vi "decade-down-counter.vi"() -> ()   [LabVIEW 2021]
uses:
  4-bit-disp.ctl
  7-segment-display.ctl
  !4-bit-cont.ctl
panel:
  out "7-segment":T1
  out "Iteration":i32
  out "!4-bit-display":T2
  out "4-bit-display":T3
  in  "Stop Button":bool
  in  "CLK":bool
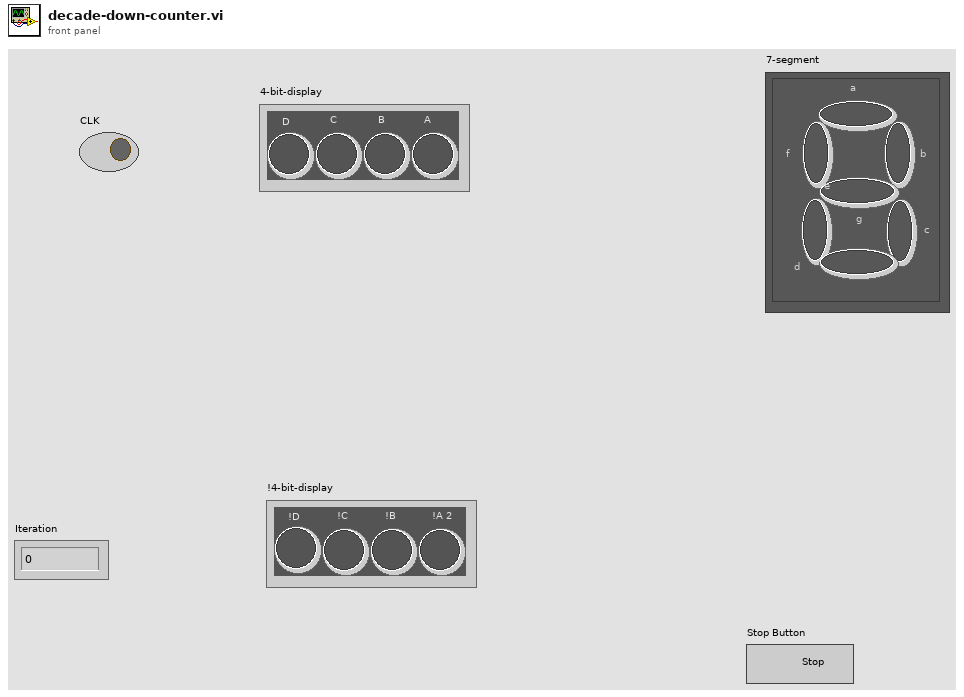
[diagram p1: front panel]
types:
  T1 = typedef "7-segment-display.ctl" = cluster{"a":bool, "b":bool, "c":bool, "d":bool, "e":bool, "f":bool, "g":bool}
  T2 = cluster{"!D":bool, "!C":bool, "!B":bool, "!A 2":bool}
  T3 = typedef "4-bit-disp.ctl" = cluster{"D":bool, "C":bool, "B":bool, "A":bool}
  T4 = typedef "!4-bit-cont.ctl" = cluster{"!D":bool, "!C":bool, "!B":bool, "!A":bool}
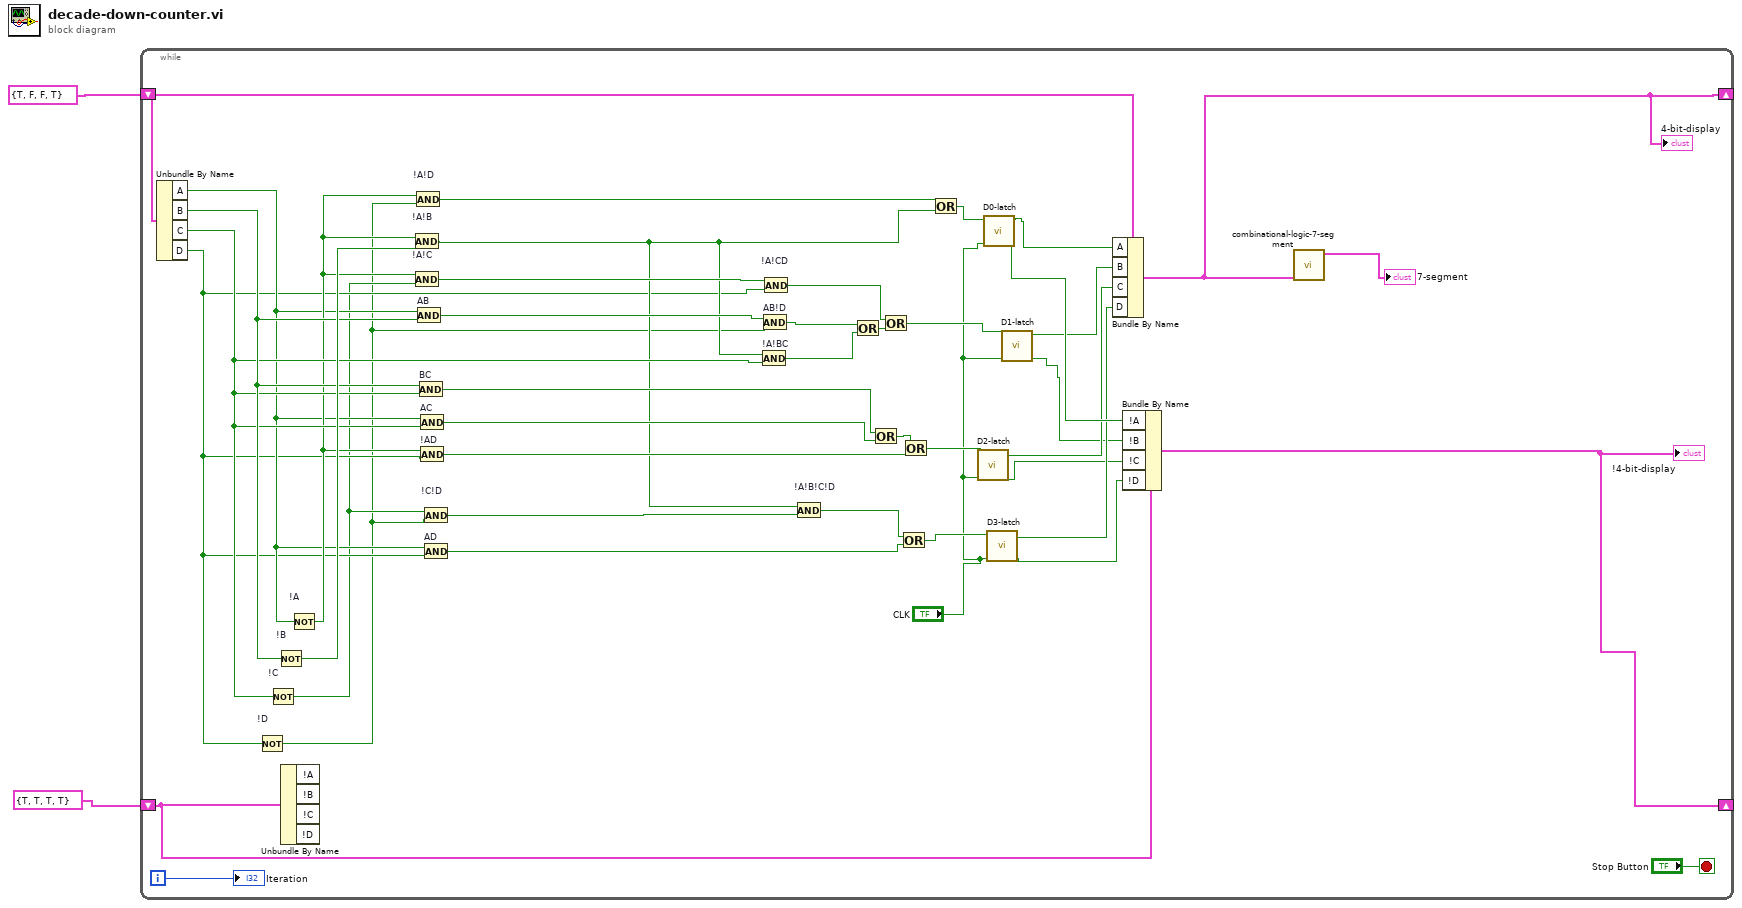
[diagram p0: block diagram]
diagram:
  n1 = while {
    shift-right: [w26] -> _
    shift-left: T3 {"D"=TRUE, "C"=FALSE, "B"=FALSE, "A"=TRUE} ("4-bit-display") -> [w44]
    shift-right: [w42] -> _
    shift-left: T4 {"!D"=TRUE, "!C"=TRUE, "!B"=TRUE, "!A"=TRUE} ("4-bit-display") -> [w43]
    i -> [w41]
    stop <- "Stop Button" stop-if-true
    n2 = Unbundle By Name(w44) -> ("A"=w6:bool, "B"=w16:bool, "C"=w15:bool, "D"=w5:bool)
    n3 = Not "!D"(x=w5) -> (.not. x?=w3:bool)
    n4 = Not "!C"(x=w15) -> (.not. x?=w4:bool)
    n5 = Not "!B"(x=w16) -> (.not. x?=w24:bool)
    n6 = Unbundle By Name(w43) -> ()  [unwired: 4 out]
    n7 = Not "!A"(x=w6) -> (.not. x?=w14:bool)
    n8 = And "!A!B"(x=w14, y=w24) -> (x .and. y?=w10:bool)
    n9 = And "!A!C"(x=w14, y=w4) -> (x .and. y?=w22:bool)
    n10 = And "!A!D"(x=w14, y=w3) -> (x .and. y?=w25:bool)
    n11 = And "AB"(x=w6, y=w16) -> (x .and. y?=w19:bool)
    n12 = And "BC"(x=w16, y=w15) -> (x .and. y?=w13:bool)
    n13 = And "AC"(x=w6, y=w15) -> (x .and. y?=w12:bool)
    n14 = And "!AD"(x=w14, y=w5) -> (x .and. y?=w11:bool)
    n15 = And "!C!D"(x=w4, y=w3) -> (x .and. y?=w9:bool)
    n16 = And "AD"(x=w6, y=w5) -> (x .and. y?=w7:bool)
    n17 = And "!A!BC"(x=w10, y=w15) -> (x .and. y?=w18:bool)
    n18 = And "AB!D"(x=w19, y=w3) -> (x .and. y?=w20:bool)
    n19 = And "!A!CD"(x=w22, y=w5) -> (x .and. y?=w23:bool)
    n20 = And "!A!B!C!D"(x=w10, y=w9) -> (x .and. y?=w8:bool)
    n21 = Or(x=w20, y=w18) -> (x .or. y?=w21:bool)
    n22 = Or(x=w13, y=w12) -> (x .or. y?=w17:bool)
    n23 = Or(x=w23, y=w21) -> (x .or. y?=w32:bool)
    n24 = Or(x=w8, y=w7) -> (x .or. y?=w36:bool)
    n25 = Or(x=w17, y=w11) -> (x .or. y?=w35:bool)
    n26 = Or(x=w25, y=w10) -> (x .or. y?=w28:bool)
    n27 = call "D2-latch.vi"("CLK"="CLK", "D"=w35) -> ("'Q"=w34:bool, "Q"=w33:bool)  [unwired: 8 in]
    n28 = call "D0-latch.vi"("CLK"="CLK", "D"=w28) -> ("'Q"=w39:bool, "Q"=w40:bool)  [unwired: 8 in]
    n29 = call "D3-latch.vi"("CLK"="CLK", "D"=w36) -> ("'Q"=w37:bool, "Q"=w38:bool)  [unwired: 8 in]
    n30 = call "D1-latch.vi"("CLK"="CLK", "D"=w32) -> ("'Q"=w31:bool, "Q"=w30:bool)  [unwired: 8 in]
    n31 = Bundle By Name(cluster=w44, "A"=w40, "B"=w30, "C"=w33, "D"=w38) -> (w26:T3)
    "4-bit-display" <- w26
    n32 = Bundle By Name(cluster=w43, "!A"=w39, "!B"=w31, "!C"=w34, "!D"=w37) -> (w42:T4)
    "!4-bit-display" <- w42
    n33 = call "combinational-logic-7-segment.vi"("4-bit-reg-input"=w26) -> ("7-segment CTRL out"=→"7-segment":T1)  [unwired: 9 in, 1 out]
    "Iteration" <- w41
  }
